vi "Memory.Pointer.Compare Contents.vi"(8 "error in (no error)":errorcluster, 10 "Pointer b in":refnum<class "Memory.Pointer.lvclass">, 11 "Pointer a in":refnum<class "Memory.Pointer.lvclass">) -> (0 "error out":errorcluster, 1 "equal contents?":bool, 2 "Pointer b out":refnum<class "Memory.Pointer.lvclass">, 3 "Pointer a out":refnum<class "Memory.Pointer.lvclass">)   [LabVIEW 2016, in "Memory.lvlib" / "Memory.Pointer.lvclass"]
uses:
  Memory.Pointer.lvclass
  Memory.Pointer.Read.1D.U8.vi
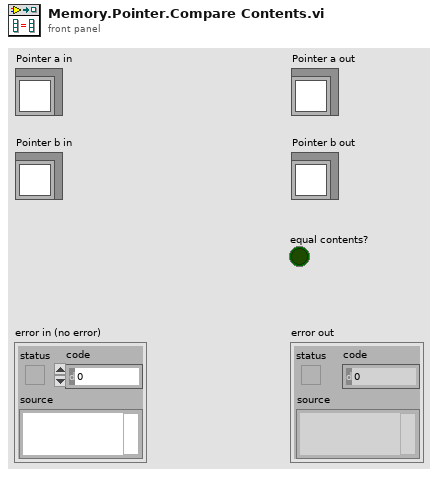
[diagram p1: front panel]
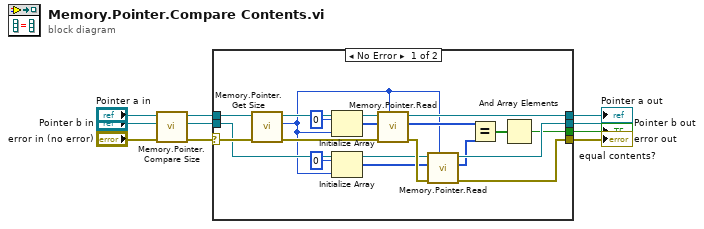
[diagram p0: block diagram]
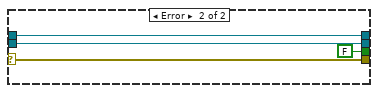
[diagram p2: hidden frame]
diagram:
  n1 = call "Memory.Pointer.Compare Size.vi"("error in (no error)"="error in (no error)", "Pointer b in"="Pointer b in", "Pointer a in"="Pointer a in") -> ("error out"=w1:errorcluster, "Pointer b out"=w4:refnum<class "Memory.Pointer.lvclass">, "Pointer a out"=w8:refnum<class "Memory.Pointer.lvclass">)  [unwired: 5 in, 1 out]
  n2 = case shown="No Error" w1 {
    selector: w1 -> [w27 w30]
    tunnel: w8 -> [w24 w29]
    tunnel: w4 -> [w22 w28]
    tunnel: [w16 w29] -> w7
    tunnel: [w14 w28] -> w6
    tunnel: [w15 w30] -> w5
    tunnel: [w12 FALSE] -> w2
    frame No Error {
      n3 = call "Memory.Pointer.Get Size.vi"("Pointer in"=w24) -> ("size"=w11:u64, "Pointer out"=w18:refnum<class "Memory.Pointer.lvclass">)  [unwired: 9 in]
      n4 = Initialize Array(u8 0 ("element"), w11) -> (w19:u8[])
      n5 = Initialize Array(u8 0 ("element"), w11) -> (w20:u8[])
      n6 = call-poly "Memory.Pointer.Read.vi"("count (-1: all)"=w11, "error in (no error)"=w27, "buffer in"=w19, "Pointer in"=w18) -> ("error out"=w23:errorcluster, "buffer out"=w21:u8[], "Pointer out"=w16:refnum<class "Memory.Pointer.lvclass">)  [unwired: 4 in, 1 out]
      n7 = call-poly "Memory.Pointer.Read.vi"("count (-1: all)"=w11, "error in (no error)"=w23, "buffer in"=w20, "Pointer in"=w22) -> ("error out"=w15:errorcluster, "buffer out"=w13:u8[], "Pointer out"=w14:refnum<class "Memory.Pointer.lvclass">)  [unwired: 4 in, 1 out]
      n8 = Equal?(x=w21, y=w13) -> (x = y?=w17:bool[])
      n9 = And Array Elements(Boolean array=w17) -> (logical AND=w12:bool)
    }
    frame Error {
    }
  }
  "error out" <- w5
  "equal contents?" <- w2
  "Pointer a out" <- w7
  "Pointer b out" <- w6
